vi "通道配置模块.vi"() -> ()   [LabVIEW 2010]
uses:
  <vilib>/Utility/file.llb/Write To Spreadsheet File (string).vi
  <vilib>/Utility/file.llb/Read From Spreadsheet File (string).vi
panel:
  in  "btn_返回":bool
  in  "选项卡控件":T1(tab)
  in  "配置文件列表1":u16(ring) items=["123.xls", "12333.xls", "1234.xls", "12345.xls", "123666.xls", "12368966.xls"]
  in  "D_IN_1":string[][](table) caption="表格"
  in  "btn_保存配置":bool
  in  "保存配置文件名称1":string
  in  "保存配置文件名称 2":string
  in  "配置文件列表2":u16(ring)
  in  "btn_保存配置 2":bool
  in  "D_IN_2":string[][](table) caption="表格"
  in  "保存配置文件名称 3":string
  in  "配置文件列表3":u16(ring)
  in  "btn_保存配置 3":bool
  in  "D_IN_3":string[][](table) caption="表格"
  in  "保存配置文件名称 4":string
  in  "配置文件列表4":u16(ring)
  in  "btn_保存配置 4":bool
  in  "D_IN_4":string[][](table) caption="表格"
  # "控制板通道及参数配置"
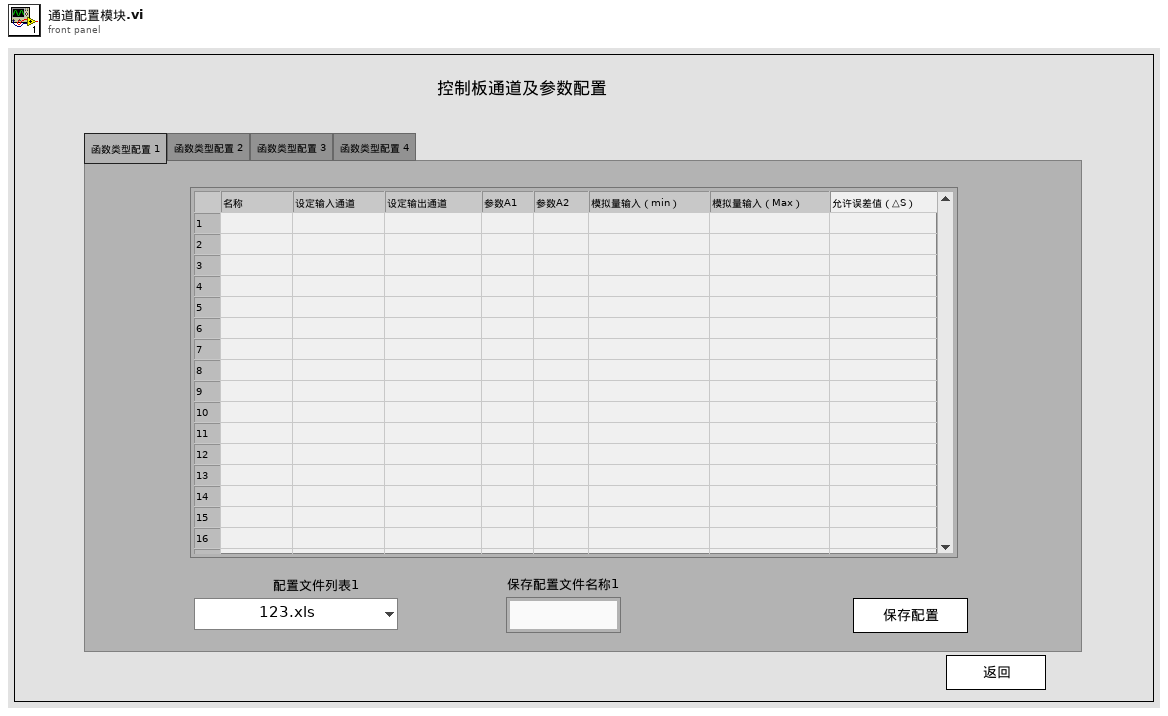
[diagram p1: front panel]
types:
  T1 = enum32{"函数类型配置 1", "函数类型配置 2", "函数类型配置 3", "函数类型配置 4"}
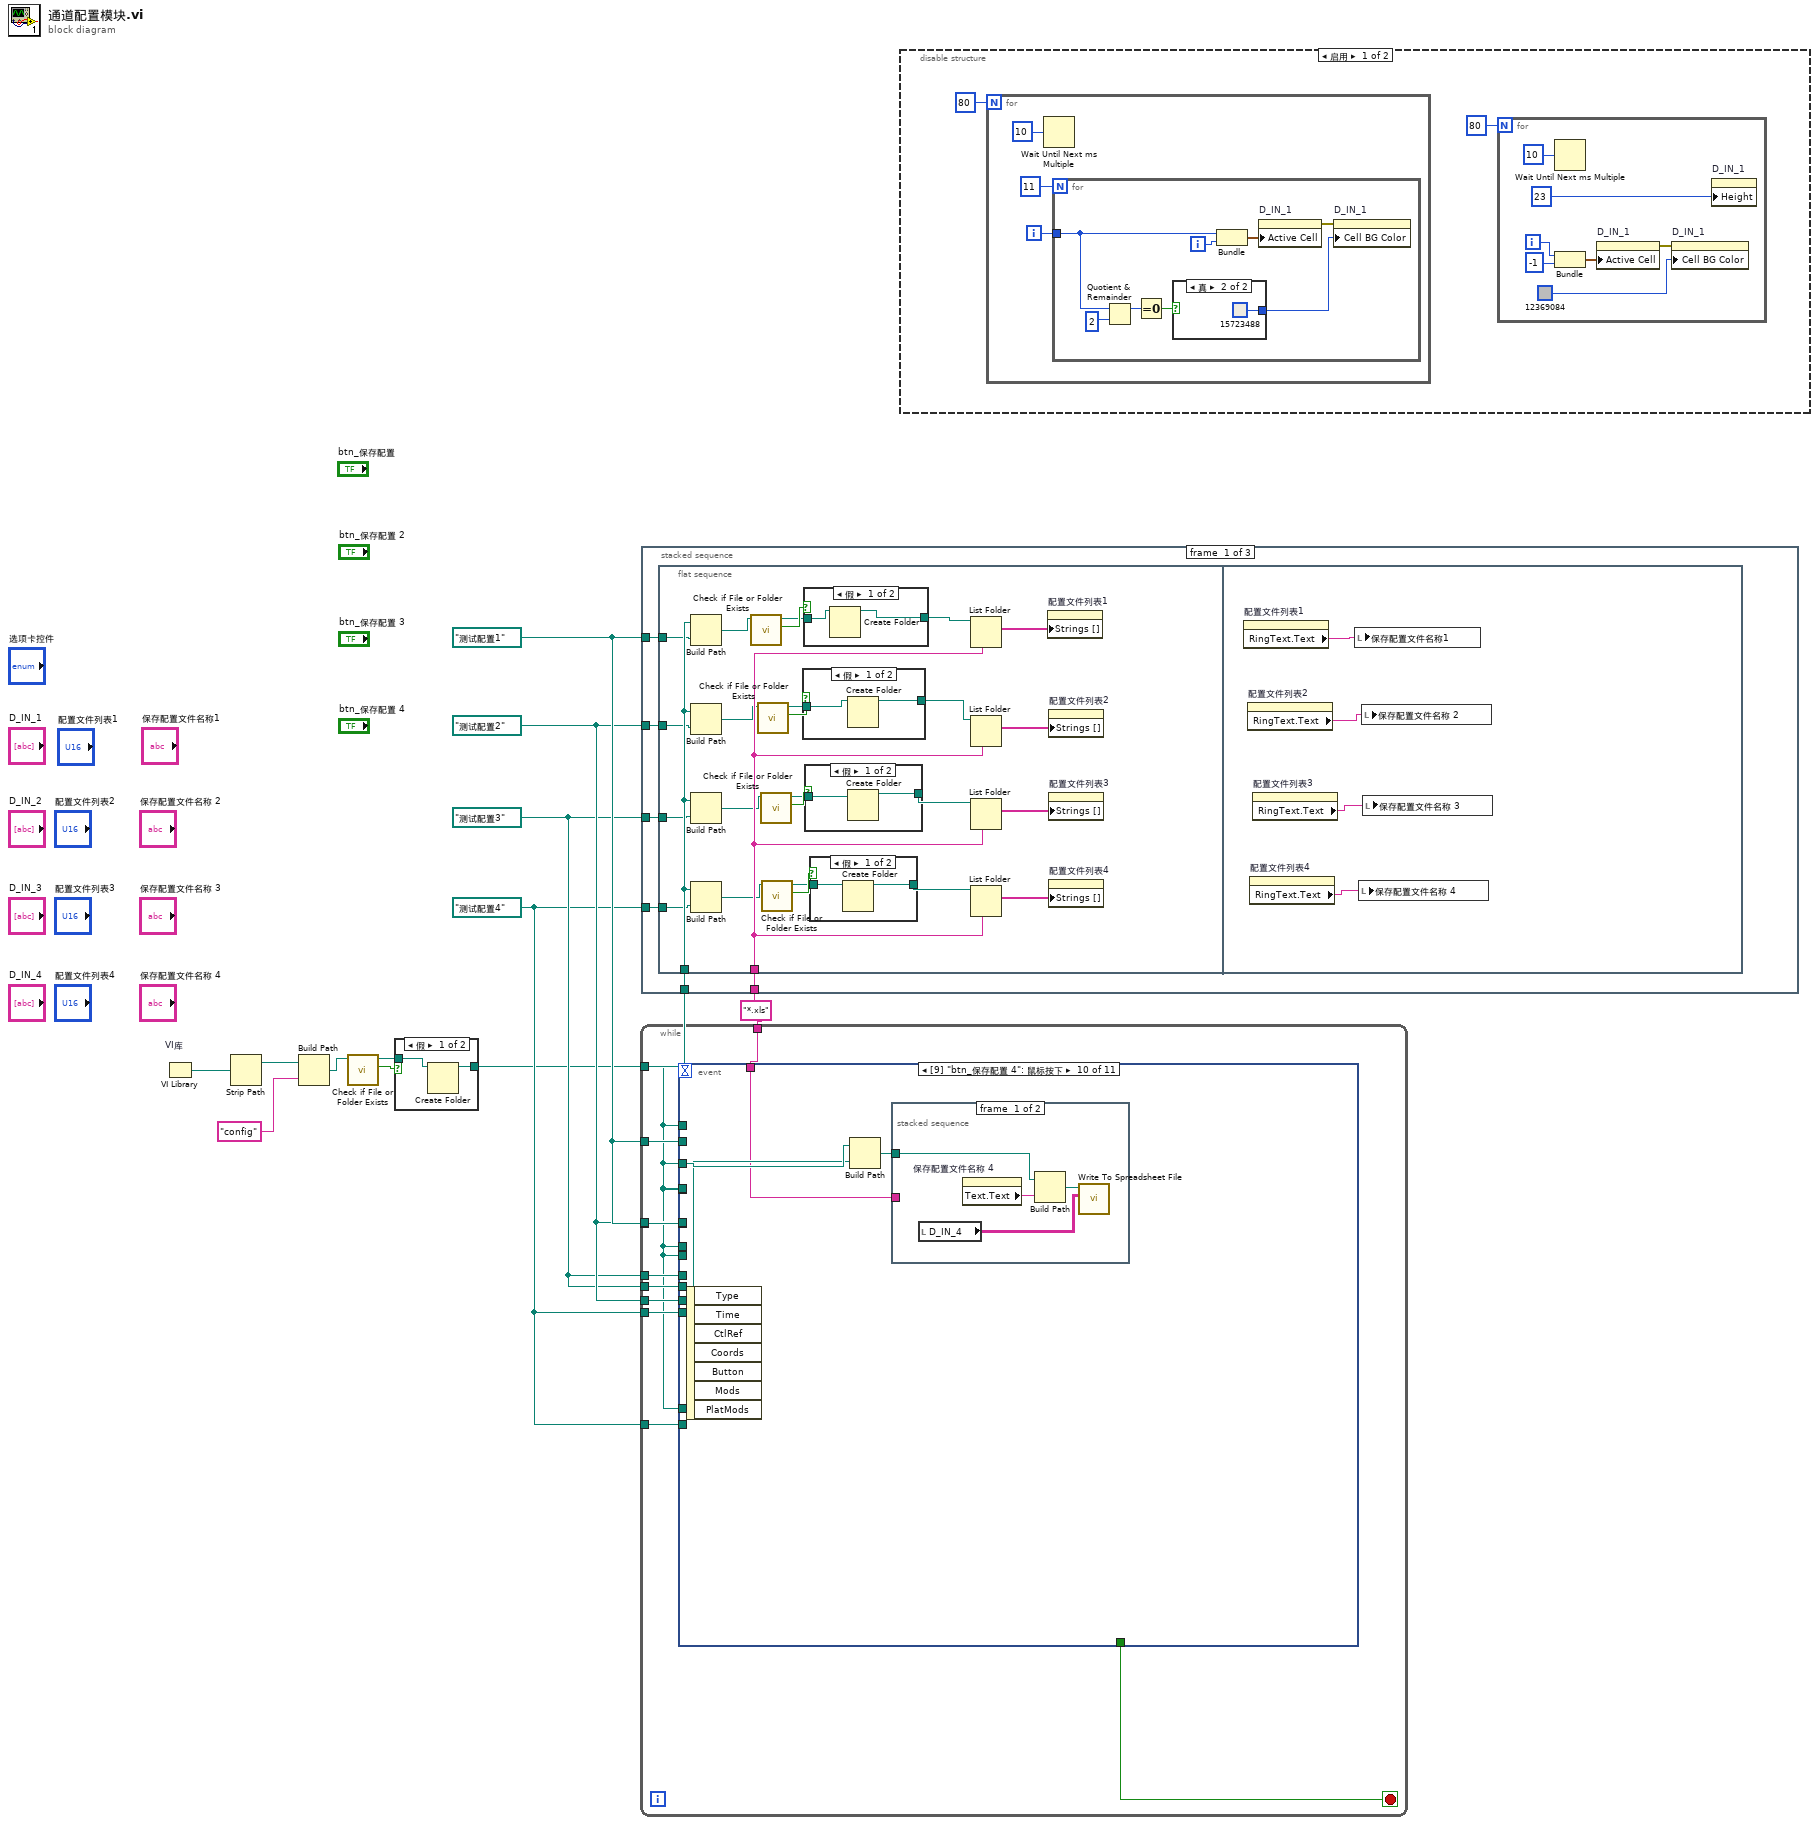
[diagram p0: block diagram]
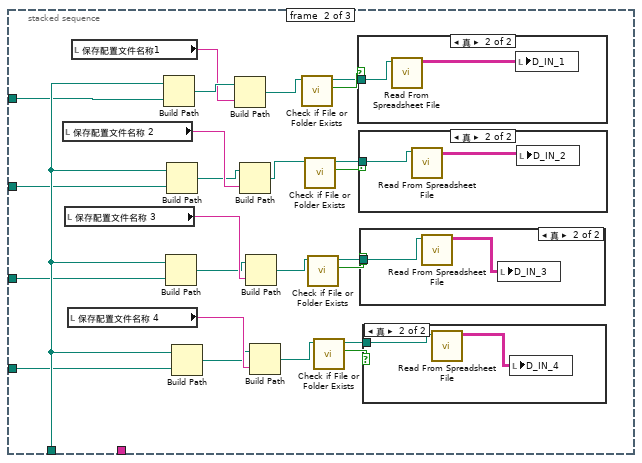
[diagram p7: hidden frame]
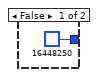
[diagram p13: hidden frame]
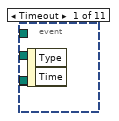
[diagram p15: hidden frame]
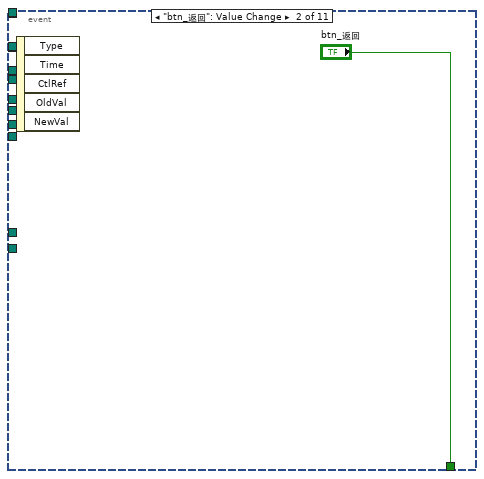
[diagram p16: hidden frame]
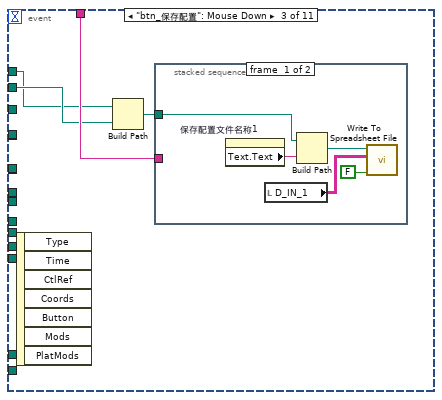
[diagram p17: hidden frame]
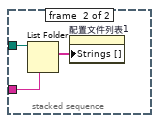
[diagram p18: hidden frame]
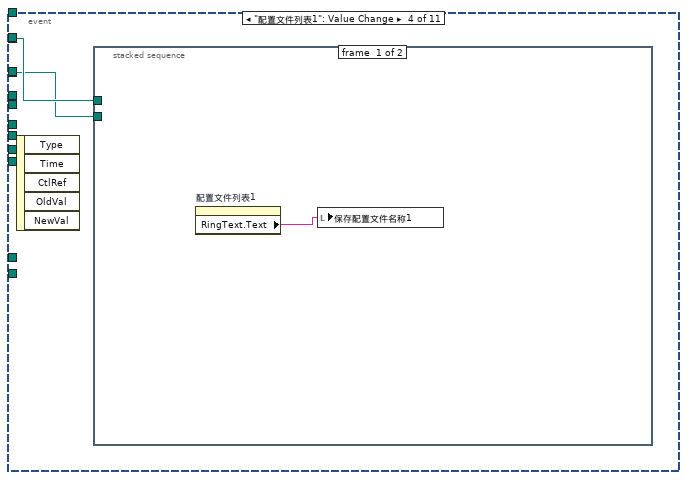
[diagram p19: hidden frame]
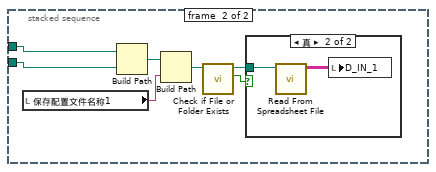
[diagram p20: hidden frame]
diagram:
  w8 = path "测试配置4"
  w9 = path "测试配置3"
  w10 = path "测试配置2"
  w11 = path "测试配置1"
  w12 = "*.xls" ("模式")
  n1 = VI Library "VI库"() -> (path=w7:path)
  n2 = Strip Path(path=w7) -> (stripped path=w6:path)  [unwired: 1 out]
  n3 = Build Path(base path=w6, name or relative path="config" ("名称或相对路径")) -> (appended path=w4:path)
  n4 = call <vilib>:"Check if File or Folder Exists.vi"("path"=w4) -> ("file or folder exists?"=w3:bool, "dup path"=w2:path)  [unwired: 8 in, 1 out]
  n5 = case shown="假" w3 {
    tunnel: w2 -> [w14 w15]
    tunnel: [w13 w15] -> w1
    frame False {
      n6 = Create Folder(path (use dialog)=w14) -> (created path=w13:path)  [unwired: 2 in, 2 out]
    }
    frame True {
    }
  }
  n7 = while {
    tunnel: w1 -> [w17]
    tunnel: w11 -> [w25]
    tunnel: w10 -> [w24]
    tunnel: w9 -> [w23]
    tunnel: w8 -> [w22]
    tunnel: w12 -> [w21]
    tunnel: w11 -> [w20]
    tunnel: w10 -> [w19]
    tunnel: w9 -> [w18]
    tunnel: w8 -> [w16]
    stop <- w26 stop-if-true
    n8 = event shown="[9] \"btn_保存配置 4\": 鼠标按下" {
      selector: _ -> [_ _ _ _ _ _ _ _ _ _ _]
      dyn-events: _ -> [_ _ _ _ _ _ _ _ _ _ _]
      timeout: _ -> [_ _ _ _ _ _ _ _ _ _ _]
      tunnel: [_ "btn_返回" _ _ _ _ _ _ _ _ TRUE] -> w26
      tunnel: w17 -> [_ _ w29 _ _ _ _ _ _ _ _]
      tunnel: w25 -> [_ _ w30 _ _ _ _ _ _ _ _]
      tunnel: w17 -> [_ _ _ _ _ _ _ w90 w102 _ _]
      tunnel: w24 -> [_ _ _ _ _ _ _ w89 _ _ _]
      tunnel: w23 -> [_ _ _ _ _ _ _ _ w101 _ _]
      tunnel: w17 -> [_ _ _ _ _ _ _ _ _ w113 _]
      tunnel: w22 -> [_ _ _ _ _ _ _ _ _ w112 _]
      tunnel: w21 -> [_ _ w31 _ _ _ _ w91 w100 w110 _]
      tunnel: w17 -> [_ _ _ w41 _ _ _ _ _ _ _]
      tunnel: w20 -> [_ _ _ w40 _ _ _ _ _ _ _]
      tunnel: w17 -> [_ _ _ _ w53 _ _ _ _ _ _]
      tunnel: w19 -> [_ _ _ _ w52 _ _ _ _ _ _]
      tunnel: w17 -> [_ _ _ _ _ w65 _ _ _ _ _]
      tunnel: w18 -> [_ _ _ _ _ w64 _ _ _ _ _]
      tunnel: w17 -> [_ _ _ _ _ _ w77 _ _ _ _]
      tunnel: w16 -> [_ _ _ _ _ _ w76 _ _ _ _]
      event Timeout {
        n9 = event-data() -> ()  [unwired: 1 in, 2 out]
      }
      event "btn_返回": Value Change {
        n10 = event-data() -> ()  [unwired: 1 in, 5 out]
      }
      event "btn_保存配置": Mouse Down {
        n11 = event-data() -> ()  [unwired: 1 in, 7 out]
        n12 = Build Path(base path=w29, name or relative path=w30) -> (appended path=w28:path)
        n13 = stacked-sequence {
          tunnel: w31 -> [_ w38]
          tunnel: w28 -> [w32 w39]
          frame #0 {
            n14 = property on="保存配置文件名称1" class="Str"() -> ("Text.Text"=w33:string)  [unwired: 2 in, 2 out]
            n15 = local read "D_IN_1"() -> (w34:string[][])
            n16 = Build Path(base path=w32, name or relative path=w33) -> (appended path=w35:path)
            n17 = call-poly <vilib>:"Write To Spreadsheet File.vi"("append to file? (new file:F)"=FALSE, "2D data"=w34, "file path (dialog if empty)"=w35) -> ()  [unwired: 5 in, 1 out]
          }
          frame #1 {
            n18 = List Folder(path=w39, pattern=w38) -> (filenames=w37:string[])  [unwired: 2 in, 3 out]
            n19 = property on="配置文件列表1" class="Ring (严格)"("Strings []"=w37) -> ()  [unwired: 2 in, 2 out]
          }
        }
      }
      event "配置文件列表1": Value Change {
        n20 = event-data() -> ()  [unwired: 1 in, 5 out]
        n21 = stacked-sequence {
          tunnel: w41 -> [_ w49]
          tunnel: w40 -> [_ w48]
          frame #0 {
            n22 = property on="配置文件列表1" class="Ring (严格)"() -> ("RingText.Text"=w42:string)  [unwired: 2 in, 2 out]
            n23 = local write "保存配置文件名称1"(w42) -> ()
          }
          frame #1 {
            n24 = local read "保存配置文件名称1"() -> (w46:string)
            n25 = Build Path(base path=w49, name or relative path=w48) -> (appended path=w47:path)
            n26 = Build Path(base path=w47, name or relative path=w46) -> (appended path=w45:path)
            n27 = call <vilib>:"Check if File or Folder Exists.vi"("path"=w45) -> ("file or folder exists?"=w44:bool, "dup path"=w43:path)  [unwired: 8 in, 1 out]
            n28 = case shown="真" w44 {
              tunnel: w43 -> [_ w51]
              frame False {
              }
              frame True {
                n29 = call-poly <vilib>:"Read From Spreadsheet File.vi"("file path (dialog if empty)"=w51) -> ("all rows"=w50:string[][])  [unwired: 6 in, 4 out]
                n30 = local write "D_IN_1"(w50) -> ()
              }
            }
          }
        }
      }
      event "配置文件列表2": Value Change {
        n31 = event-data() -> ()  [unwired: 1 in, 5 out]
        n32 = stacked-sequence {
          tunnel: w53 -> [_ w58]
          tunnel: w52 -> [_ w57]
          frame #0 {
            n33 = property on="配置文件列表2" class="Ring (严格)"() -> ("RingText.Text"=w54:string)  [unwired: 2 in, 2 out]
            n34 = local write "保存配置文件名称 2"(w54) -> ()
          }
          frame #1 {
            n35 = local read "保存配置文件名称 2"() -> (w55:string)
            n36 = Build Path(base path=w58, name or relative path=w57) -> (appended path=w56:path)
            n37 = Build Path(base path=w56, name or relative path=w55) -> (appended path=w60:path)
            n38 = call <vilib>:"Check if File or Folder Exists.vi"("path"=w60) -> ("file or folder exists?"=w61:bool, "dup path"=w59:path)  [unwired: 8 in, 1 out]
            n39 = case shown="真" w61 {
              tunnel: w59 -> [_ w63]
              frame False {
              }
              frame True {
                n40 = call-poly <vilib>:"Read From Spreadsheet File.vi"("file path (dialog if empty)"=w63) -> ("all rows"=w62:string[][])  [unwired: 6 in, 4 out]
                n41 = local write "D_IN_2"(w62) -> ()
              }
            }
          }
        }
      }
      event "配置文件列表3": Value Change {
        n42 = event-data() -> ()  [unwired: 1 in, 5 out]
        n43 = stacked-sequence {
          tunnel: w65 -> [_ w73]
          tunnel: w64 -> [_ w71]
          frame #0 {
            n44 = property on="配置文件列表3" class="Ring (严格)"() -> ("RingText.Text"=w66:string)  [unwired: 2 in, 2 out]
            n45 = local write "保存配置文件名称 3"(w66) -> ()
          }
          frame #1 {
            n46 = local read "保存配置文件名称 3"() -> (w70:string)
            n47 = Build Path(base path=w73, name or relative path=w71) -> (appended path=w72:path)
            n48 = Build Path(base path=w72, name or relative path=w70) -> (appended path=w69:path)
            n49 = call <vilib>:"Check if File or Folder Exists.vi"("path"=w69) -> ("file or folder exists?"=w68:bool, "dup path"=w67:path)  [unwired: 8 in, 1 out]
            n50 = case shown="真" w68 {
              tunnel: w67 -> [_ w74]
              frame False {
              }
              frame True {
                n51 = call-poly <vilib>:"Read From Spreadsheet File.vi"("file path (dialog if empty)"=w74) -> ("all rows"=w75:string[][])  [unwired: 6 in, 4 out]
                n52 = local write "D_IN_3"(w75) -> ()
              }
            }
          }
        }
      }
      event "配置文件列表4": Value Change {
        n53 = event-data() -> ()  [unwired: 1 in, 5 out]
        n54 = stacked-sequence {
          tunnel: w77 -> [_ w85]
          tunnel: w76 -> [_ w84]
          frame #0 {
            n55 = property on="配置文件列表4" class="Ring (严格)"() -> ("RingText.Text"=w78:string)  [unwired: 2 in, 2 out]
            n56 = local write "保存配置文件名称 4"(w78) -> ()
          }
          frame #1 {
            n57 = local read "保存配置文件名称 4"() -> (w82:string)
            n58 = Build Path(base path=w85, name or relative path=w84) -> (appended path=w83:path)
            n59 = Build Path(base path=w83, name or relative path=w82) -> (appended path=w81:path)
            n60 = call <vilib>:"Check if File or Folder Exists.vi"("path"=w81) -> ("file or folder exists?"=w80:bool, "dup path"=w79:path)  [unwired: 8 in, 1 out]
            n61 = case shown="真" w80 {
              tunnel: w79 -> [_ w86]
              frame False {
              }
              frame True {
                n62 = call-poly <vilib>:"Read From Spreadsheet File.vi"("file path (dialog if empty)"=w86) -> ("all rows"=w87:string[][])  [unwired: 6 in, 4 out]
                n63 = local write "D_IN_4"(w87) -> ()
              }
            }
          }
        }
      }
      event "btn_保存配置 2": Mouse Down {
        n64 = event-data() -> ()  [unwired: 1 in, 7 out]
        n65 = Build Path(base path=w90, name or relative path=w89) -> (appended path=w88:path)
        n66 = stacked-sequence {
          tunnel: w91 -> [_ w97]
          tunnel: w88 -> [w93 w98]
          frame #0 {
            n67 = local read "D_IN_2"() -> (w94:string[][])
            n68 = property on="保存配置文件名称 2" class="Str"() -> ("Text.Text"=w92:string)  [unwired: 2 in, 2 out]
            n69 = Build Path(base path=w93, name or relative path=w92) -> (appended path=w95:path)
            n70 = call-poly <vilib>:"Write To Spreadsheet File.vi"("2D data"=w94, "file path (dialog if empty)"=w95) -> ()  [unwired: 6 in, 1 out]
          }
          frame #1 {
            n71 = List Folder(path=w98, pattern=w97) -> (filenames=w96:string[])  [unwired: 2 in, 3 out]
            n72 = property on="配置文件列表2" class="Ring (严格)"("Strings []"=w96) -> ()  [unwired: 2 in, 2 out]
          }
        }
      }
      event "btn_保存配置 3": Mouse Down {
        n73 = event-data() -> ()  [unwired: 1 in, 7 out]
        n74 = Build Path(base path=w102, name or relative path=w101) -> (appended path=w99:path)
        n75 = stacked-sequence {
          tunnel: w100 -> [_ w108]
          tunnel: w99 -> [w104 w109]
          frame #0 {
            n76 = local read "D_IN_3"() -> (w105:string[][])
            n77 = property on="保存配置文件名称 3" class="Str"() -> ("Text.Text"=w103:string)  [unwired: 2 in, 2 out]
            n78 = Build Path(base path=w104, name or relative path=w103) -> (appended path=w106:path)
            n79 = call-poly <vilib>:"Write To Spreadsheet File.vi"("2D data"=w105, "file path (dialog if empty)"=w106) -> ()  [unwired: 6 in, 1 out]
          }
          frame #1 {
            n80 = List Folder(path=w109, pattern=w108) -> (filenames=w107:string[])  [unwired: 2 in, 3 out]
            n81 = property on="配置文件列表3" class="Ring (严格)"("Strings []"=w107) -> ()  [unwired: 2 in, 2 out]
          }
        }
      }
      event "btn_保存配置 4": Mouse Down {
        n82 = event-data() -> ()  [unwired: 1 in, 7 out]
        n83 = Build Path(base path=w113, name or relative path=w112) -> (appended path=w111:path)
        n84 = stacked-sequence {
          tunnel: w111 -> [w115 w120]
          tunnel: w110 -> [_ w119]
          frame #0 {
            n85 = local read "D_IN_4"() -> (w116:string[][])
            n86 = property on="保存配置文件名称 4" class="Str"() -> ("Text.Text"=w114:string)  [unwired: 2 in, 2 out]
            n87 = Build Path(base path=w115, name or relative path=w114) -> (appended path=w117:path)
            n88 = call-poly <vilib>:"Write To Spreadsheet File.vi"("2D data"=w116, "file path (dialog if empty)"=w117) -> ()  [unwired: 6 in, 1 out]
          }
          frame #1 {
            n89 = List Folder(path=w120, pattern=w119) -> (filenames=w118:string[])  [unwired: 2 in, 3 out]
            n90 = property on="配置文件列表4" class="Ring (严格)"("Strings []"=w118) -> ()  [unwired: 2 in, 2 out]
          }
        }
      }
      event Panel Close {
        n91 = event-data() -> ()  [unwired: 1 in, 3 out]
      }
    }
  }
  n92 = stacked-sequence {
    tunnel: w1 -> [w127 w191 _]
    tunnel: w8 -> [w126 w184 _]
    tunnel: w9 -> [w125 w188 _]
    tunnel: w10 -> [w124 w189 _]
    tunnel: w11 -> [w123 w190 _]
    tunnel: w12 -> [w122 _ _]
    frame #0 {
      n93 = flat-sequence {
        tunnel: w127 -> [w149]
        tunnel: w126 -> [w148]
        tunnel: w125 -> [w147]
        tunnel: w124 -> [w146]
        tunnel: w123 -> [w145]
        tunnel: w122 -> [w144]
        frame #0 {
          n94 = Build Path(base path=w149, name or relative path=w145) -> (appended path=w143:path)
          n95 = Build Path(base path=w149, name or relative path=w146) -> (appended path=w139:path)
          n96 = Build Path(base path=w149, name or relative path=w147) -> (appended path=w135:path)
          n97 = Build Path(base path=w149, name or relative path=w148) -> (appended path=w131:path)
          n98 = call <vilib>:"Check if File or Folder Exists.vi"("path"=w143) -> ("file or folder exists?"=w142:bool, "dup path"=w141:path)  [unwired: 8 in, 1 out]
          n99 = call <vilib>:"Check if File or Folder Exists.vi"("path"=w139) -> ("file or folder exists?"=w138:bool, "dup path"=w137:path)  [unwired: 8 in, 1 out]
          n100 = call <vilib>:"Check if File or Folder Exists.vi"("path"=w135) -> ("file or folder exists?"=w134:bool, "dup path"=w133:path)  [unwired: 8 in, 1 out]
          n101 = call <vilib>:"Check if File or Folder Exists.vi"("path"=w131) -> ("file or folder exists?"=w130:bool, "dup path"=w129:path)  [unwired: 8 in, 1 out]
          n102 = case shown="假" w138 {
            tunnel: w137 -> [w161 w162]
            tunnel: [w160 w162] -> w136
            frame False {
              n103 = Create Folder(path (use dialog)=w161) -> (created path=w160:path)  [unwired: 2 in, 2 out]
            }
            frame True {
            }
          }
          n104 = case shown="假" w142 {
            tunnel: w141 -> [w164 w165]
            tunnel: [w163 w165] -> w140
            frame False {
              n105 = Create Folder(path (use dialog)=w164) -> (created path=w163:path)  [unwired: 2 in, 2 out]
            }
            frame True {
            }
          }
          n106 = case shown="假" w134 {
            tunnel: w133 -> [w158 w159]
            tunnel: [w157 w159] -> w132
            frame False {
              n107 = Create Folder(path (use dialog)=w158) -> (created path=w157:path)  [unwired: 2 in, 2 out]
            }
            frame True {
            }
          }
          n108 = case shown="假" w130 {
            tunnel: w129 -> [w155 w156]
            tunnel: [w154 w156] -> w128
            frame False {
              n109 = Create Folder(path (use dialog)=w155) -> (created path=w154:path)  [unwired: 2 in, 2 out]
            }
            frame True {
            }
          }
          n110 = List Folder(path=w140, pattern=w144) -> (filenames=w150:string[])  [unwired: 2 in, 3 out]
          n111 = List Folder(path=w136, pattern=w144) -> (filenames=w153:string[])  [unwired: 2 in, 3 out]
          n112 = List Folder(path=w132, pattern=w144) -> (filenames=w152:string[])  [unwired: 2 in, 3 out]
          n113 = List Folder(path=w128, pattern=w144) -> (filenames=w151:string[])  [unwired: 2 in, 3 out]
          n114 = property on="配置文件列表1" class="Ring (严格)"("Strings []"=w150) -> ()  [unwired: 2 in, 2 out]
          n115 = property on="配置文件列表2" class="Ring (严格)"("Strings []"=w153) -> ()  [unwired: 2 in, 2 out]
          n116 = property on="配置文件列表3" class="Ring (严格)"("Strings []"=w152) -> ()  [unwired: 2 in, 2 out]
          n117 = property on="配置文件列表4" class="Ring (严格)"("Strings []"=w151) -> ()  [unwired: 2 in, 2 out]
        }
        frame #1 {
          n118 = property on="配置文件列表1" class="Ring (严格)"() -> ("RingText.Text"=w169:string)  [unwired: 2 in, 2 out]
          n119 = property on="配置文件列表2" class="Ring (严格)"() -> ("RingText.Text"=w166:string)  [unwired: 2 in, 2 out]
          n120 = property on="配置文件列表4" class="Ring (严格)"() -> ("RingText.Text"=w167:string)  [unwired: 2 in, 2 out]
          n121 = property on="配置文件列表3" class="Ring (严格)"() -> ("RingText.Text"=w168:string)  [unwired: 2 in, 2 out]
          n122 = local write "保存配置文件名称1"(w169) -> ()
          n123 = local write "保存配置文件名称 4"(w167) -> ()
          n124 = local write "保存配置文件名称 2"(w166) -> ()
          n125 = local write "保存配置文件名称 3"(w168) -> ()
        }
      }
    }
    frame #1 {
      n126 = local read "保存配置文件名称 2"() -> (w192:string)
      n127 = local read "保存配置文件名称 3"() -> (w187:string)
      n128 = local read "保存配置文件名称 4"() -> (w183:string)
      n129 = local read "保存配置文件名称1"() -> (w193:string)
      n130 = Build Path(base path=w191, name or relative path=w190) -> (appended path=w194:path)
      n131 = Build Path(base path=w191, name or relative path=w188) -> (appended path=w186:path)
      n132 = Build Path(base path=w191, name or relative path=w189) -> (appended path=w185:path)
      n133 = Build Path(base path=w191, name or relative path=w184) -> (appended path=w182:path)
      n134 = Build Path(base path=w194, name or relative path=w193) -> (appended path=w181:path)
      n135 = Build Path(base path=w185, name or relative path=w192) -> (appended path=w179:path)
      n136 = Build Path(base path=w186, name or relative path=w187) -> (appended path=w175:path)
      n137 = Build Path(base path=w182, name or relative path=w183) -> (appended path=w172:path)
      n138 = call <vilib>:"Check if File or Folder Exists.vi"("path"=w181) -> ("file or folder exists?"=w180:bool, "dup path"=w176:path)  [unwired: 8 in, 1 out]
      n139 = call <vilib>:"Check if File or Folder Exists.vi"("path"=w179) -> ("file or folder exists?"=w178:bool, "dup path"=w177:path)  [unwired: 8 in, 1 out]
      n140 = call <vilib>:"Check if File or Folder Exists.vi"("path"=w175) -> ("file or folder exists?"=w174:bool, "dup path"=w173:path)  [unwired: 8 in, 1 out]
      n141 = call <vilib>:"Check if File or Folder Exists.vi"("path"=w172) -> ("file or folder exists?"=w171:bool, "dup path"=w170:path)  [unwired: 8 in, 1 out]
      n142 = case shown="真" w180 {
        tunnel: w176 -> [_ w201]
        frame False {
        }
        frame True {
          n143 = call-poly <vilib>:"Read From Spreadsheet File.vi"("file path (dialog if empty)"=w201) -> ("all rows"=w202:string[][])  [unwired: 6 in, 4 out]
          n144 = local write "D_IN_1"(w202) -> ()
        }
      }
      n145 = case shown="真" w178 {
        tunnel: w177 -> [_ w199]
        frame False {
        }
        frame True {
          n146 = call-poly <vilib>:"Read From Spreadsheet File.vi"("file path (dialog if empty)"=w199) -> ("all rows"=w200:string[][])  [unwired: 6 in, 4 out]
          n147 = local write "D_IN_2"(w200) -> ()
        }
      }
      n148 = case shown="真" w174 {
        tunnel: w173 -> [_ w197]
        frame False {
        }
        frame True {
          n149 = call-poly <vilib>:"Read From Spreadsheet File.vi"("file path (dialog if empty)"=w197) -> ("all rows"=w198:string[][])  [unwired: 6 in, 4 out]
          n150 = local write "D_IN_3"(w198) -> ()
        }
      }
      n151 = case shown="真" w171 {
        tunnel: w170 -> [_ w195]
        frame False {
        }
        frame True {
          n152 = call-poly <vilib>:"Read From Spreadsheet File.vi"("file path (dialog if empty)"=w195) -> ("all rows"=w196:string[][])  [unwired: 6 in, 4 out]
          n153 = local write "D_IN_4"(w196) -> ()
        }
      }
    }
    frame #2 {
    }
  }
  n154 = disable-structure shown="启用" {
    frame Enabled {
      n155 = for {
        N: 80 -> [_]
        i -> [w206]
        n156 = Wait Until Next ms Multiple(millisecond multiple=u32 10 ("毫秒倍数")) -> ()  [unwired: 1 out]
        n157 = for {
          N: 11 -> [_]
          tunnel: w206 -> [w214]
          i -> [w211]
          n158 = Quotient & Remainder(x=w214, y=2) -> (x-y*floor(x/y)=w212:i32)  [unwired: 1 out]
          n159 = Equal To 0?(x=w212) -> (x = 0?=w215:bool)
          n160 = case shown="真" w215 {
            tunnel: [u32 16448250 u32 15723488] -> w209
            frame False {
            }
            frame True {
            }
          }
          n161 = Bundle(w214, w211) -> (w210:cluster{i32, i32})  [unwired: 1 in]
          n162 = property on="D_IN_1" class="Tbl (严格)"("Active Cell"=w210) -> (error out=w208:errorcluster)  [unwired: 2 in, 1 out]
          n163 = property on="D_IN_1" class="Tbl (严格)"(error in=w208, "Cell BG Color"=w209) -> ()  [unwired: 1 in, 2 out]
        }
      }
      n164 = for {
        N: 80 -> [_]
        i -> [w223]
        n165 = Wait Until Next ms Multiple(millisecond multiple=u32 10 ("毫秒倍数")) -> ()  [unwired: 1 out]
        n166 = Bundle(w223, "y"=-1) -> (w222:cluster{i32, "y":i32})  [unwired: 1 in]
        n167 = property on="D_IN_1" class="Tbl (严格)"("Active Cell"=w222) -> (error out=w221:errorcluster)  [unwired: 2 in, 1 out]
        n168 = property on="D_IN_1" class="Tbl (严格)"(error in=w221, "Cell BG Color"=u32 12369084) -> ()  [unwired: 1 in, 2 out]
        n169 = property on="D_IN_1" class="Tbl (严格)"("Height"=u32 23 ("XControl:容器边界:高度")) -> ()  [unwired: 2 in, 2 out]
      }
    }
    frame Disabled {
    }
  }
